vi "Split WAVEFORM array in half.vi"(11 "AO Array":waveform(dbl)[](array[waveform])) -> (2 "Array":waveform(dbl)[](array[waveform]), 3 "Array 2":waveform(dbl)[](array[waveform]))   [LabVIEW 2016, in "lockin.lvclass"]
uses:
  lockin.lvclass
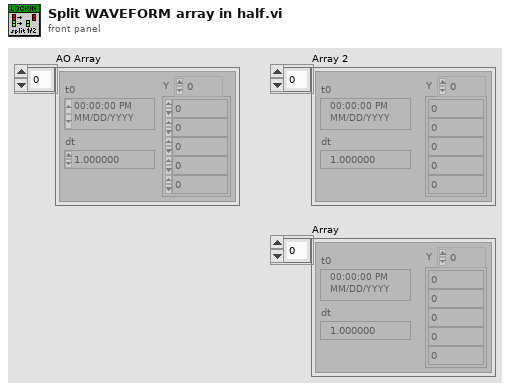
[diagram p1: front panel]
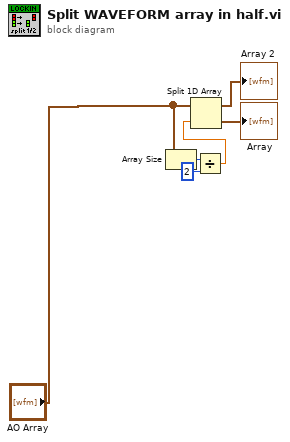
[diagram p0: block diagram]
diagram:
  n1 = Array Size(array="AO Array") -> (size(s)=w3:i32)
  n2 = Divide(x=w3, y=2) -> (x/y=w5:dbl)
  n3 = Split 1D Array(array="AO Array", index=w5) -> (first subarray=→"Array 2":waveform(dbl)[], second subarray=→"Array":waveform(dbl)[])
